vi "ReadSingleJoint.vi"(0 "node":string, 1 "Angle Name":T1(ring)) -> (2 "Position":dbl, 3 "Velocity":dbl, 4 "Effort":dbl)   [LabVIEW 2010]
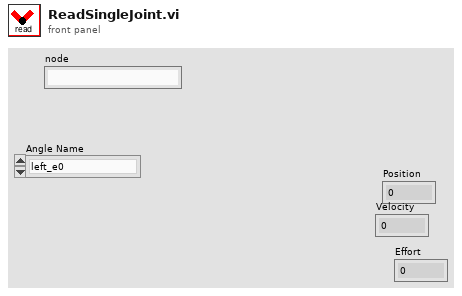
[diagram p1: front panel]
types:
  T1 = enum16{"left_e0", "left_e1", "left_s0", "left_s1", "left_w0", "left_w1", "left_w2", "right_e0", "right_e1", "right_s0", "right_s1", "right_w0", "right_w1", "right_w2"}
  T2 = cluster{"Joint Name":string, "Position":dbl, "Velocity":dbl, "Effort":dbl}[]
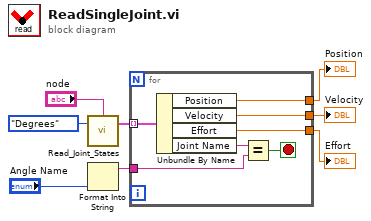
[diagram p0: block diagram]
diagram:
  n1 = call "Read_Joint_States.vi"("Units (deg)"=enum16{"Radians", "Degrees"}."Degrees", "node"="node") -> ("Joint States"=w6:T2)  [unwired: 1 in, 1 out]
  n2 = Format Into String("Angle Name") -> (resulting string=w8:string)  [unwired: 3 in, 1 out]
  n3 = for {
    tunnel: w6 -> [w15] mode=indexing
    tunnel: w8 -> [w13]
    tunnel: [w11] -> w2
    tunnel: [w10] -> w3
    tunnel: [w9] -> w4
    stop <- w12 stop-if-true
    n4 = Unbundle By Name(w15) -> ("Position"=w11:dbl, "Velocity"=w10:dbl, "Effort"=w9:dbl, "Joint Name"=w14:string)
    n5 = Equal?(x=w14, y=w13) -> (x = y?=w12:bool)
  }
  "Velocity" <- w3
  "Position" <- w2
  "Effort" <- w4
